vi "DialogPrompt.vi"(10 "Dialog prompt":string) -> (1 "OK out":bool, 2 "Usert Txt(out)":string)   [LabVIEW 2010]
panel:
  in  "Cancel":bool
  in  "OK Button":bool
  in  "Usert Txt":string
  out "String":string
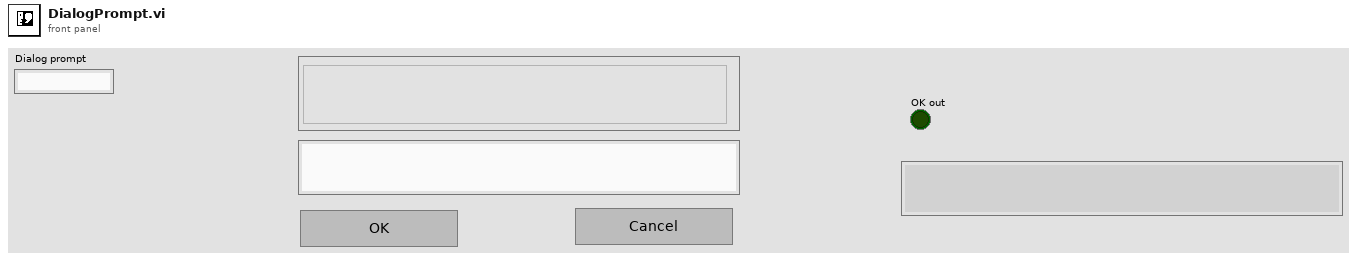
[diagram p1: front panel]
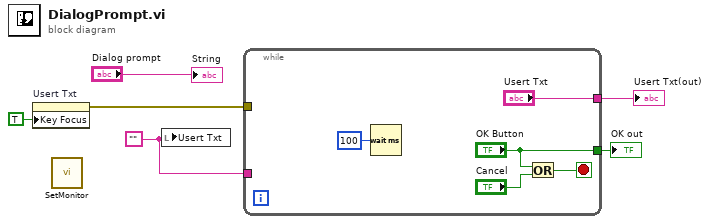
[diagram p0: block diagram]
diagram:
  w3 = ""
  n1 = property on="Usert Txt" class="Str"("Key Focus"=TRUE) -> (error out=w2:errorcluster)  [unwired: 2 in, 1 out]
  n2 = call "SetMonitor.vi"() -> ()  [unwired: 10 in, 2 out]
  n3 = local write "Usert Txt"(w3) -> ()
  n4 = while {
    tunnel: ["OK Button"] -> w5
    tunnel: ["Usert Txt"] -> w4
    tunnel: w3 -> [_]
    tunnel: w2 -> [_]
    stop <- w11 stop-if-true
    n5 = Wait (ms)(milliseconds to wait=u32 100) -> ()  [unwired: 1 out]
    n6 = Or(x="OK Button", y="Cancel") -> (x .or. y?=w11:bool)
  }
  "OK out" <- w5
  "Usert Txt(out)" <- w4
  "String" <- "Dialog prompt"
